vi "onOwnershipChanged.vi"(8 "error in":errorcluster, 11 "SMO.ErrorInjection in":refnum<class "SMO.ErrorInjection.lvclass">) -> (0 "error out":errorcluster, 3 "SMO.ErrorInjection out":refnum<class "SMO.ErrorInjection.lvclass">)   [LabVIEW 2013, in "SMO.ErrorInjection.lvclass"]
uses:
  SMO.ErrorInjection.lvclass
  src/SMO/SMO.lvclass
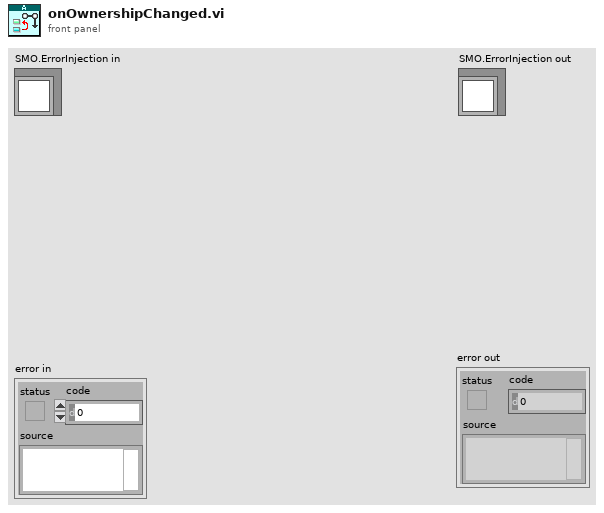
[diagram p1: front panel]
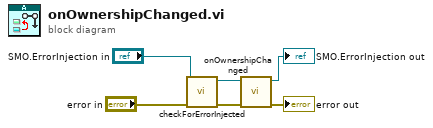
[diagram p0: block diagram]
diagram:
  n1 = call "checkForErrorInjected.vi"("error in (no error)"="error in", "SMO.ErrorInjection in"="SMO.ErrorInjection in") -> ("error out"=w3:errorcluster, "SMO.ErrorInjection dup"=w1:refnum<class "SMO.ErrorInjection.lvclass">)  [unwired: 8 in]
  n2 = call-parent "onOwnershipChanged.vi"("error in"=w3, "SMO in"=w1) -> ("error out"=→"error out":errorcluster, "SMO out"=→"SMO.ErrorInjection out":refnum<class "SMO.ErrorInjection.lvclass">)  [unwired: 8 in]
